vi "T7 Strm Config Compare KAG.vi"(1 "Strm Config 1":T1={"Scan Rate (Hz)"=1000.0, "Samples Per Packet"=512, "Resolution Index"=0, "Buffer Size (bytes)"=32768, "NumScans"=1500, "Read Timeout (ms)"=5000, "Scan Table"=[{"Channel"=0, "BipGain"=0, "Input Config"="Single-Ended"}, {"Channel"=1, "BipGain"=0, "Input Config"="Single-Ended"}, {"Channel"=2, "BipGain"=0, "Input Config"="Single-Ended"}, {"Channel"=3, "BipGain"=0, "Input Config"="Single-Ended"}]} {"Samples Per Packet" max=512 step=1; "Buffer Size (bytes)" max=32768 step=1; "Resolution Index" max=8 step=1; "Scan Rate (Hz)" max=100000; "Scan Table"."BipGain" items=["x1", "x10", "x100", "x1000"]; "Scan Table"."Channel" step=1}, 2 "Strm Config 2":T1={"Scan Rate (Hz)"=1000.0, "Samples Per Packet"=512, "Resolution Index"=0, "Buffer Size (bytes)"=32768, "NumScans"=1500, "Read Timeout (ms)"=5000, "Scan Table"=[{"Channel"=0, "BipGain"=0, "Input Config"="Single-Ended"}, {"Channel"=1, "BipGain"=0, "Input Config"="Single-Ended"}, {"Channel"=2, "BipGain"=0, "Input Config"="Single-Ended"}, {"Channel"=3, "BipGain"=0, "Input Config"="Single-Ended"}]} {"Samples Per Packet" max=512 step=1; "Buffer Size (bytes)" max=32768 step=1; "Resolution Index" max=8 step=1; "Scan Rate (Hz)" max=100000; "Scan Table"."BipGain" items=["x1", "x10", "x100", "x1000"]; "Scan Table"."Channel" step=1}) -> (0 "result":bool)   [LabVIEW 2022 SP3]
uses:
  T7 Stream Config KAG.ctl
panel:
  out "Scan Table Size":bool
  out "Config":bool
  out "Gain":bool
  out "AIN#":bool
  out "NumScans":bool
  out "Scan Rate (Hz)":bool
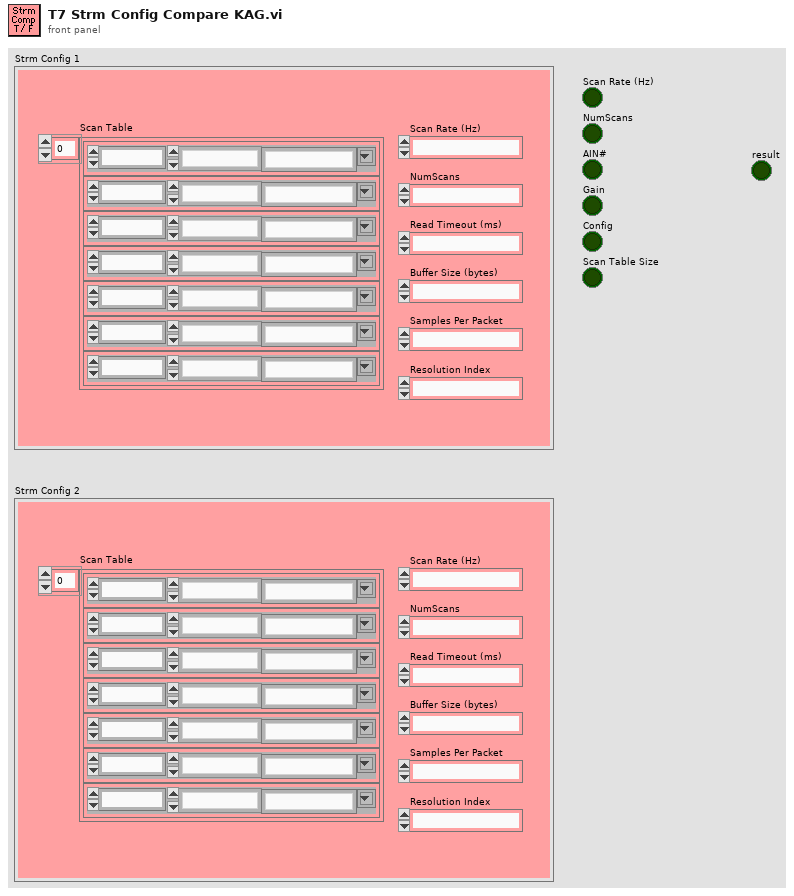
[diagram p1: front panel]
types:
  T1 = typedef "T7 Stream Config KAG.ctl" = cluster{"Scan Rate (Hz)":sgl, "Samples Per Packet":u32, "Resolution Index":u32, "Buffer Size (bytes)":u32, "NumScans":u32, "Read Timeout (ms)":u32, "Scan Table":cluster{"Channel":u32, "BipGain":u32, "Input Config":string}[]}
  T2 = cluster{"Channel":u32, "BipGain":u32, "Input Config":string}[]
  T3 = cluster{"Scan Rate (Hz)":sgl, "NumScans":u32, "Scan Table":cluster{"Channel":u32, "BipGain":u32, "Input Config":string}[]}
  T4 = cluster{"Scan Rate (Hz)":bool, "NumScans":bool, "Scan Table":cluster{"Channel":bool, "BipGain":bool, "Input Config":bool}[]}
  T5 = cluster{"Channel":bool, "BipGain":bool, "Input Config":bool}[]
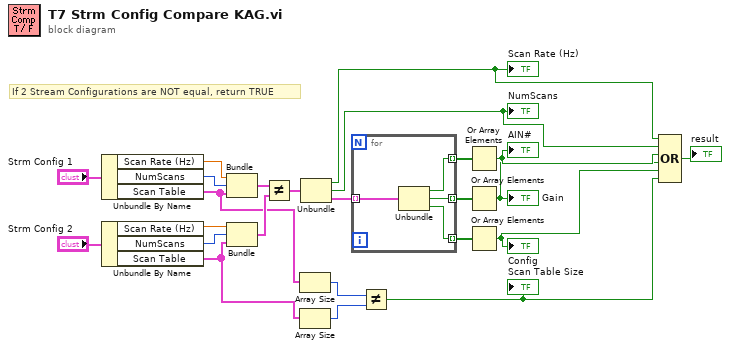
[diagram p0: block diagram]
diagram:
  # "If 2 Stream Configurations are NOT equal, return TRUE"
  n1 = Unbundle By Name("Strm Config 1") -> ("Scan Rate (Hz)"=w24:sgl, "NumScans"=w23:u32, "Scan Table"=w5:T2)
  n2 = Unbundle By Name("Strm Config 2") -> ("Scan Rate (Hz)"=w20:sgl, "NumScans"=w19:u32, "Scan Table"=w4:T2)
  n3 = Bundle("Scan Rate (Hz)"=w24, "NumScans"=w23, "Scan Table"=w5) -> (w22:T3)  [unwired: 1 in]
  n4 = Bundle("Scan Rate (Hz)"=w20, "NumScans"=w19, "Scan Table"=w4) -> (w18:T3)  [unwired: 1 in]
  n5 = Not Equal?(x=w22, y=w18) -> (x != y?=w17:T4)
  n6 = Array Size(array=w5) -> (size(s)=w3:i32)
  n7 = Array Size(array=w4) -> (size(s)=w2:i32)
  n8 = Unbundle(w17) -> ("Scan Rate (Hz)"=w11:bool, "NumScans"=w10:bool, "Scan Table"=w15:T5)
  "Scan Rate (Hz)" <- w11
  "NumScans" <- w10
  n9 = for {
    tunnel: w15 -> [w28] mode=indexing
    tunnel: [w27] -> w14 mode=indexing
    tunnel: [w26] -> w13 mode=indexing
    tunnel: [w25] -> w12 mode=indexing
    n10 = Unbundle(w28) -> ("Channel"=w27:bool, "BipGain"=w26:bool, "Input Config"=w25:bool)
  }
  n11 = Not Equal?(x=w3, y=w2) -> (x != y?=w1:bool)
  "Scan Table Size" <- w1
  n12 = Or Array Elements(Boolean array=w14) -> (logical OR=w9:bool)
  "AIN#" <- w9
  n13 = Or Array Elements(Boolean array=w13) -> (logical OR=w8:bool)
  "Gain" <- w8
  n14 = Or Array Elements(Boolean array=w12) -> (logical OR=w7:bool)
  "Config" <- w7
  n15 = Compound Arithmetic op=OR(w11, w10, w9, w8, w7, w1) -> (→"result":bool)
